vi "WLAN_FrameCapture.vi"(7 "error in (no error)":errorcluster, 9 "Trigger level":dbl format="%0.2f", 10 "session handle":refnum<k15>) -> ()   [LabVIEW 2022 SP3]
uses:
  <instrlib>/niUSRP/niUSRP Fetch Rx Data (CDB Cluster).vi
  <vilib>/Analysis/NI_AALPro.lvlib
panel:
  out "error out":errorcluster
  out "x <= y?":bool
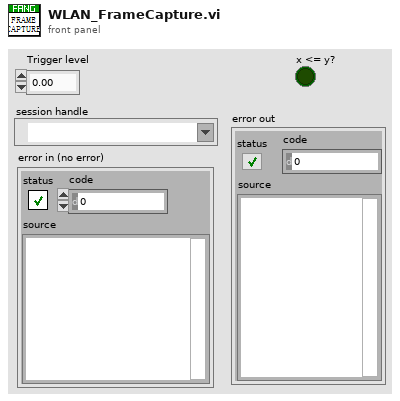
[diagram p1: front panel]
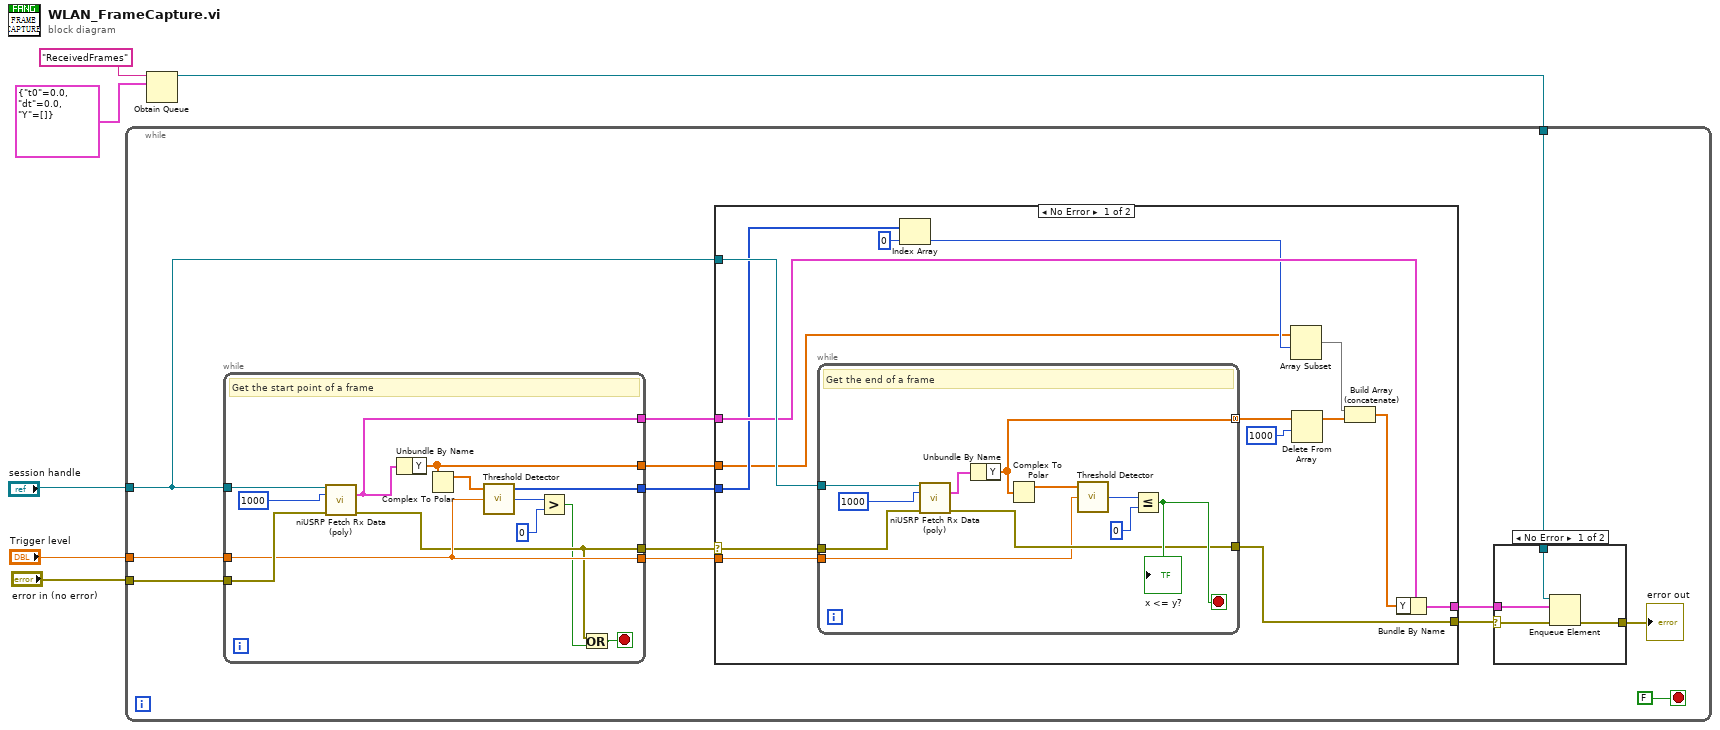
[diagram p0: block diagram]
diagram:
  n1 = Obtain Queue(name (unnamed)="ReceivedFrames", element data type=cluster{"t0":dbl, "dt":dbl, "Y":cdb[]} {"t0"=0.0, "dt"=0.0, "Y"=[]} ("data")) -> (queue out=w1:refnum<queue>)  [unwired: 3 in, 2 out]
  n2 = while {
    tunnel: "error in (no error)" -> [w19]
    tunnel: "Trigger level" -> [w18]
    tunnel: "session handle" -> [w17]
    tunnel: w1 -> [w12]
    stop <- FALSE stop-if-true
    n3 = while {
      tunnel: w17 -> [w62]
      tunnel: w19 -> [w65]
      tunnel: w18 -> [w60]
      tunnel: [w56] -> w13
      tunnel: [w60] -> w16
      tunnel: [w57] -> w15
      tunnel: [w58] -> w14
      tunnel: [w53] -> w7
      stop <- w54 stop-if-true
      # "Get the start point of a frame"
      n4 = call-poly <instrlib>:"niUSRP Fetch Rx Data (poly).vi"("session handle"=w62, "number of samples"=i64 1000, "error in (no error)"=w65) -> ("data"=w57:cluster{"t0":dbl, "dt":dbl, "Y":cdb[]}, "error out"=w56:errorcluster)  [unwired: 9 in, 2 out]
      n5 = Unbundle By Name(w57) -> ("Y"=w53:cdb[])
      n6 = Complex To Polar(r * e^(i*theta)=w53) -> (r=w59:dbl[])  [unwired: 1 out]
      n7 = call <vilib>:"Threshold Detector.vi"("threshold"=w60, "X"=w59) -> ("count"=w64:i32, "Indices"=w58:i32[])  [unwired: 1 in, 1 out]
      n8 = Greater?(x=w64, y=0) -> (0:w55:bool)
      n9 = Or(x=w56, y=w55) -> (x .or. y?=w54:bool)
    }
    n10 = case shown="No Error" w13 {
      selector: w13 -> [w29 w51]
      tunnel: w17 -> [w39 _]
      tunnel: [w38 w51] -> w10
      tunnel: w16 -> [w37 _]
      tunnel: w15 -> [w36 w52]
      tunnel: [w35 w52] -> w11
      tunnel: w14 -> [w32 _]
      tunnel: w7 -> [w25 _]
      frame No Error {
        n11 = while {
          tunnel: w39 -> [w48]
          tunnel: [w45] -> w38
          tunnel: w29 -> [w44]
          tunnel: w37 -> [w43]
          tunnel: [w40] -> w34 mode=concatenating
          stop <- w46 stop-if-true
          # "Get the end of a frame"
          n12 = call-poly <instrlib>:"niUSRP Fetch Rx Data (poly).vi"("session handle"=w48, "number of samples"=i64 1000, "error in (no error)"=w44) -> ("data"=w41:cluster{"t0":dbl, "dt":dbl, "Y":cdb[]}, "error out"=w45:errorcluster)  [unwired: 9 in, 2 out]
          n13 = Unbundle By Name(w41) -> ("Y"=w40:cdb[])
          n14 = Complex To Polar(r * e^(i*theta)=w40) -> (r=w42:dbl[])  [unwired: 1 out]
          n15 = call <vilib>:"Threshold Detector.vi"("threshold"=w43, "X"=w42) -> ("count"=w50:i32)  [unwired: 1 in, 2 out]
          n16 = Less Or Equal?(x=w50, y=0) -> (x <= y?=w46:bool)
          "x <= y?" <- w46
        }
        n17 = Index Array(array=w32, index=0) -> (element=w30:i32)
        n18 = Array Subset(array=w25, index=w30) -> (w28:cdb[])  [unwired: 1 in]
        n19 = Delete From Array(array=w34, length=1000) -> (array with subset deleted=w26:cdb[])  [unwired: 1 in, 1 out]
        n20 = Build Array (concatenate)(w28, w26) -> (w27:cdb[])
        n21 = Bundle By Name(cluster=w36, "Y"=w27) -> (w35:cluster{"t0":dbl, "dt":dbl, "Y":cdb[]})
      }
      frame Error {
      }
    }
    n22 = case shown="No Error" w10 {
      selector: w10 -> [w21 w24]
      tunnel: w12 -> [w23 _]
      tunnel: w11 -> [w22 _]
      tunnel: [w20 w24] -> w9
      frame No Error {
        n23 = Enqueue Element(queue=w23, element=w22, error in (no error)=w21) -> (error out=w20:errorcluster)  [unwired: 1 in, 2 out]
      }
      frame Error {
      }
    }
    "error out" <- w9
  }
